vi "ReadConfig.vi"() -> (0 "External Settings":T3)   [LabVIEW 2011]
uses:
  <vilib>/Utility/config.llb/Read Key (I32).vi
  <vilib>/Utility/config.llb/Read Key (U32).vi
  <vilib>/Utility/config.llb/Read Key (String).vi
  <vilib>/Utility/config.llb/Read Key (Path).vi
  <vilib>/Utility/config.llb/NI_LVConfig.lvlib
panel:
  out "Digital Multimeter Card":T1
  out "Matrix version":cluster{"Matrix version":string}
  out "Matrix version":string
  out "Components list":string
  out "Components type":T2
  out "Components type":string
  out "Digital Multimeter":T1
  out "USB Interface":T1
  out "Digital Osciliscope":T1
  out "DC Power Supply":T1
  out "Function Generator":T1
  out "Log":cluster{"Log Level":u32, "Log File":path}
  out "Log File":path
  out "Log Level":u32
  out "Oscilloscope":T4
  out "Global":T5
  out "Timeout":u32
  out "Port":i32
  out "Maximum Delay":i32
  out "Reset Time":i32
  out "Digital Multimeter":T6
  out "Powerline Frequency":u32
  out "Instrument Adress":T7
  out "4072":string
  out "USB":string
  out "5112":string
  out "4110":string
  out "5402":string
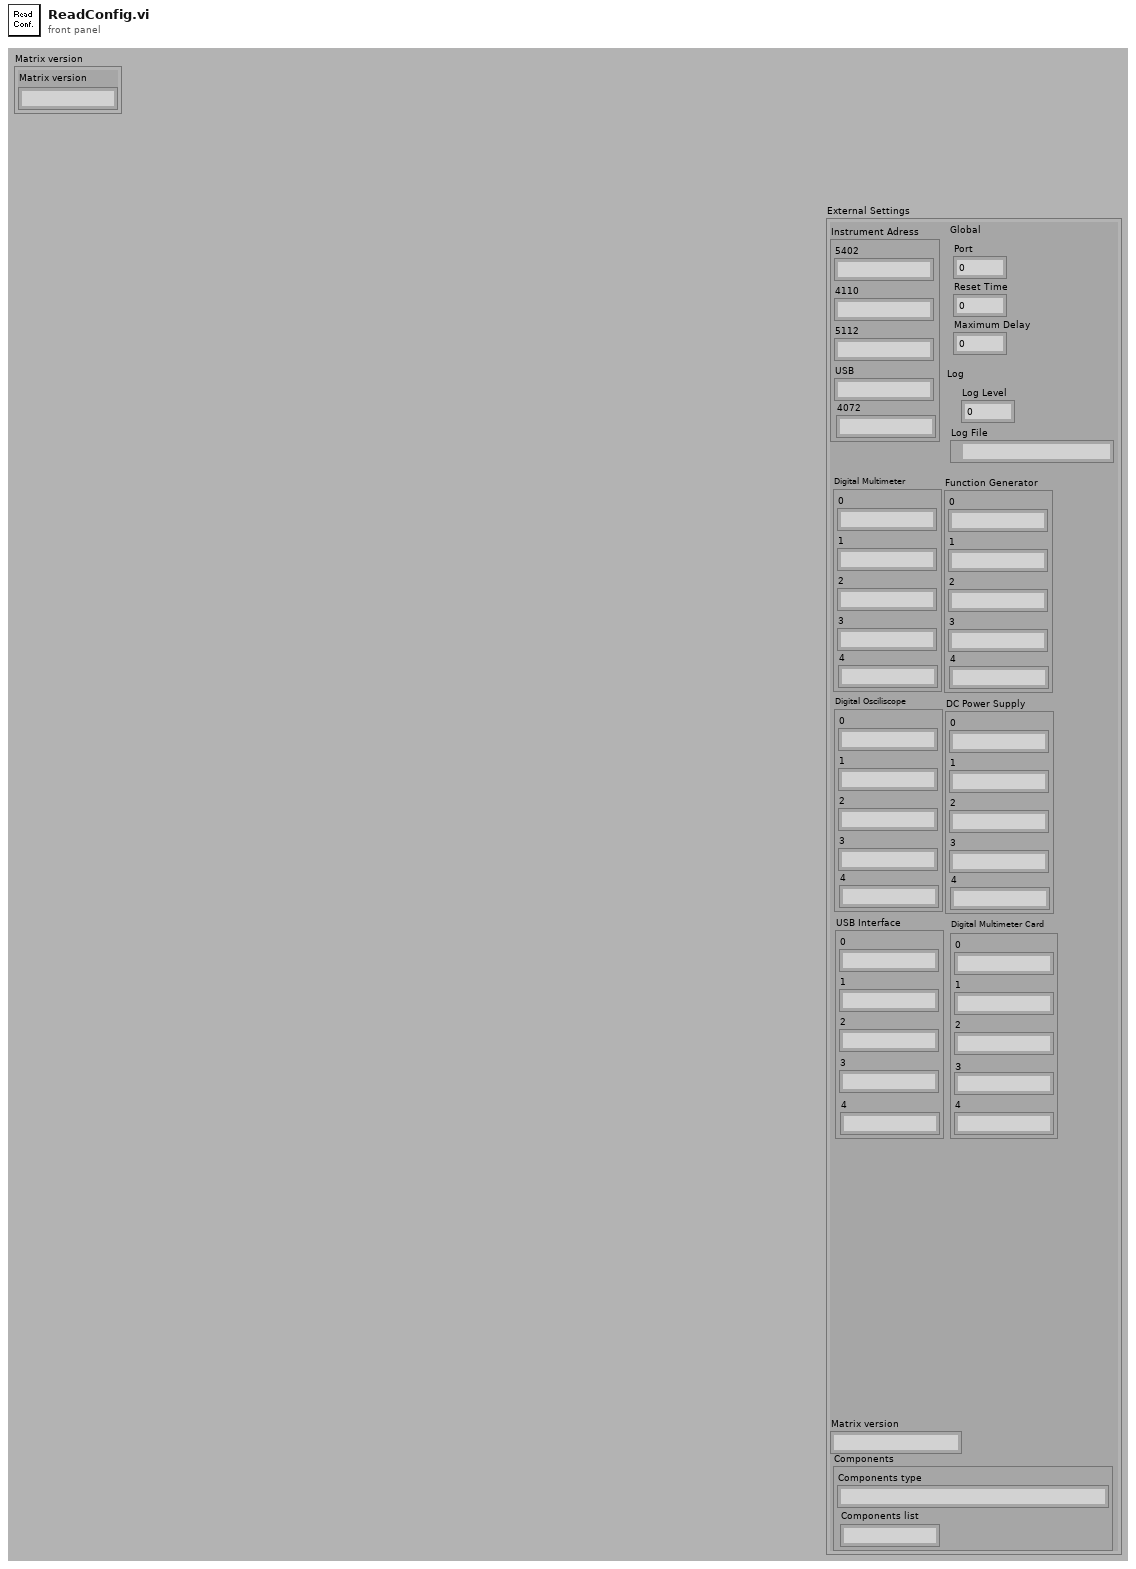
[diagram p1: front panel]
types:
  T1 = cluster{"0":string, "1":string, "2":string, "3":string, "4":string}
  T2 = cluster{"Components type":string, "Components list":string}
  T3 = cluster{"Global":cluster{"Port":i32, "Reset Time":i32, "Maximum Delay":i32}, "Instrument Adress":cluster{"5402":string, "4110":string, "5112":string, "USB":string, "4072":string}, "Log":cluster{"Log Level":u32, "Log File":path}, "Digital Multimeter":cluster{"0":string, "1":string, "2":string, "3":string, "4":string}, "Function Generator":cluster{"0":string, "1":string, "2":string, "3":string, "4":string}, "Digital Osciliscope":cluster{"0":string, "1":string, "2":string, "3":string, "4":string}, "DC Power Supply":cluster{"0":string, "1":string, "2":string, "3":string, "4":string}, "USB Interface":cluster{"0":string, "1":string, "2":string, "3":string, "4":string}, "Components":cluster{"Components type":string, "Components list":string}, "Matrix version":string, "Digital Multimeter Card 2":cluster{"0":string, "1":string, "2":string, "3":string, "4":string}}
  T4 = cluster{"Oscilloscope Board A\nResouce name":string, "Oscilloscope Board B\nResouce name":string, "Additonal Slave Trigger Delay":dbl}
  T5 = cluster{"Port":i32, "Reset Time":i32, "Maximum Delay":i32}
  T6 = cluster{"Powerline Frequency":u32, "Numeric":dbl}
  T7 = cluster{"5401":string, "4110":string, "5112":string, "USB":string, "4072":string}
  T8 = typedef "NI_LVConfig.lvlib/Config Data RefNum.ctl" = refnum<k1>
  T9 = cluster{"[0]":string, "[1]":string, "[2]":string, "[3]":string, "[4]":string}
  T10 = cluster{"Powerline Frequency":u32, "Timeout":u32}
  T11 = cluster{"5402":string, "4110":string, "5112":string, "USB":string, "4072":string}
  T12 = cluster{"Global":cluster{"Port":i32, "Reset Time":i32, "Maximum Delay":i32}, "Instrument Adress":cluster{"5401":string, "4110":string, "5112":string, "USB":string, "4072":string}, "Log":cluster{"Log Level":u32, "Log File":path}, "Digital Multimeter":cluster{"0":string, "1":string, "2":string, "3":string, "4":string}, "Function Generator":cluster{"0":string, "1":string, "2":string, "3":string, "4":string}, "Digital Osciliscope":cluster{"0":string, "1":string, "2":string, "3":string, "4":string}, "DC Power Supply":cluster{"0":string, "1":string, "2":string, "3":string, "4":string}, "USB Interface":cluster{"0":string, "1":string, "2":string, "3":string, "4":string}, "Components type":cluster{"Components type":string, "Components list":string}, "Matrix version":string, "Digital Multimeter Card":cluster{"0":string, "1":string, "2":string, "3":string, "4":string}}
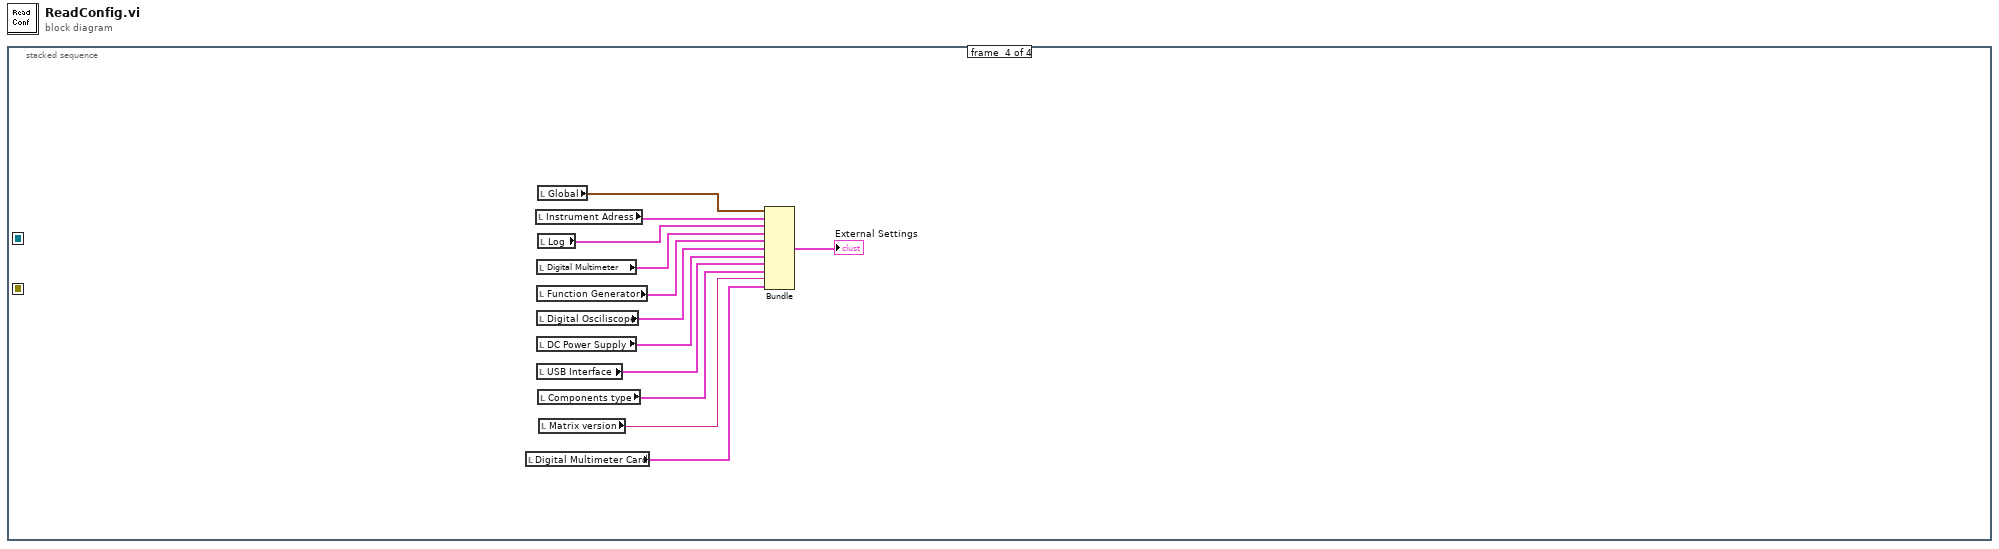
[diagram p0: block diagram]
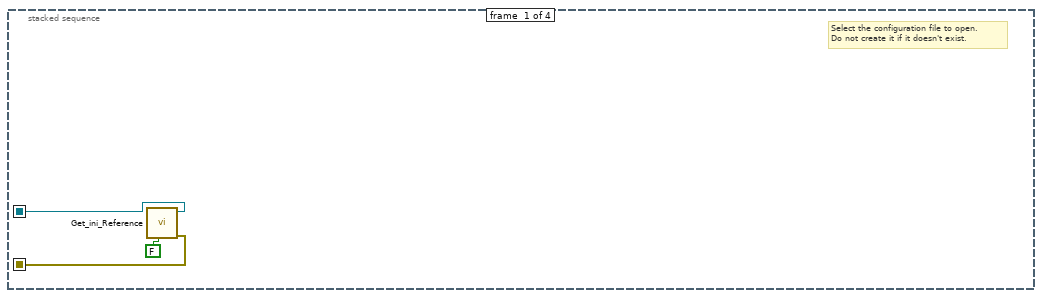
[diagram p2: hidden frame]
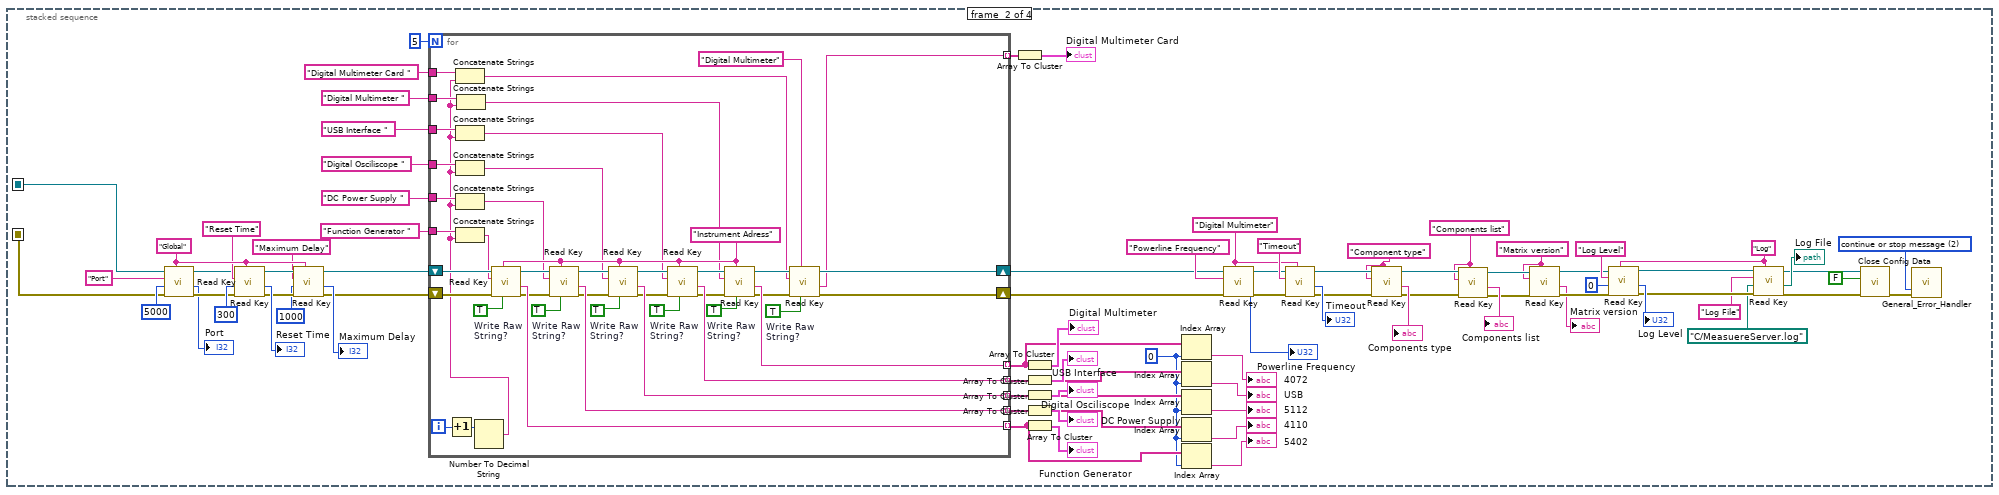
[diagram p3: hidden frame]
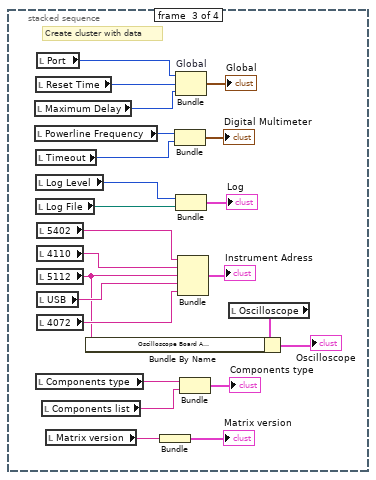
[diagram p4: hidden frame]
diagram:
  n1 = stacked-sequence {
    seq-local: [w2 _ _ _] -> [_ w56 _ _]
    seq-local: [w1 _ _ _] -> [_ w55 _ _]
    frame #0 {
      # "Select the configuration file to open.\nDo not create it if it doesn't exist."
      n2 = call "Get_ini_Reference.vi"("create file if necessary? (T)"=FALSE) -> ("Error out"=w2:errorcluster, "ini Ref"=w1:T8)  [unwired: 8 in, 1 out]
    }
    frame #1 {
      w8 = "Matrix version"
      w10 = "Components list"
      w9 = "Component type"
      w26 = 0
      w46 = "Log"
      w52 = u16 2 items=["no dialog", "OK message", "continue or stop message"] ("type of dialog (OK msg:1)")
      w78 = "Digital Multimeter" ("section")
      w74 = "Global" ("section")
      n3 = call-poly <vilib>:"Read Key.vi"("section"=w74, "error in (no error)"=w56, "default value"=u32 5000, "key"="Port" ("Key 1"), "refnum"=w55) -> ("error out"=w67:errorcluster, "value"=→"Port":i32, "refnum out"=w66:T8)  [unwired: 3 in, 1 out]
      n4 = call-poly <vilib>:"Read Key.vi"("section"=w74, "error in (no error)"=w67, "default value"=300, "key"="Reset Time", "refnum"=w66) -> ("error out"=w73:errorcluster, "value"=→"Reset Time":i32, "refnum out"=w70:T8)  [unwired: 3 in, 1 out]
      n5 = call-poly <vilib>:"Read Key.vi"("section"=w74, "error in (no error)"=w73, "default value"=1000, "key"="Maximum Delay", "refnum"=w70) -> ("error out"=w72:errorcluster, "value"=→"Maximum Delay":i32, "refnum out"=w71:T8)  [unwired: 3 in, 1 out]
      n6 = for {
        N: 5 -> [_]
        tunnel: "Digital Osciliscope " -> [w101]
        tunnel: [w123] -> w31 mode=indexing
        tunnel: [w122] -> w30 mode=indexing
        tunnel: [w121] -> w29 mode=indexing
        tunnel: [w120] -> w28 mode=indexing
        tunnel: [w119] -> w27 mode=indexing
        tunnel: "Digital Multimeter " -> [w105]
        tunnel: "Function Generator " -> [w97]
        tunnel: "DC Power Supply " -> [w100]
        tunnel: "USB Interface " -> [w104]
        shift-right: [w93] -> w39
        shift-left: w72 -> [w126]
        shift-right: [w91] -> w38
        shift-left: w71 -> [w125]
        tunnel: "Digital Multimeter Card " ("section") -> [w87]
        tunnel: [w84] -> w5 mode=indexing
        i -> [w96]
        w90 = TRUE  # Write Raw String?
        w114 = TRUE  # Write Raw String?
        w113 = TRUE  # Write Raw String?
        w112 = TRUE  # Write Raw String?
        w109 = TRUE  # Write Raw String?
        w108 = TRUE  # Write Raw String?
        w124 = "Instrument Adress" ("section")
        n7 = Increment(x=w96) -> (x+1=w95:i32)
        n8 = Number To Decimal String(number=w95) -> (decimal integer string=w88:string)  [unwired: 1 in]
        n9 = Concatenate Strings(w87, w88) -> (w86:string)
        n10 = Concatenate Strings(w104, w88) -> (w103:string)
        n11 = Concatenate Strings(w101, w88) -> (w102:string)
        n12 = Concatenate Strings(w100, w88) -> (w99:string)
        n13 = Concatenate Strings(w97, w88) -> (w98:string)
        n14 = Concatenate Strings(w105, w88) -> (w89:string)
        n15 = call-poly <vilib>:"Read Key.vi"("read raw string? (F)"=w109, "section"=w124, "error in (no error)"=w126, "key"=w98, "refnum"=w125) -> ("error out"=w106:errorcluster, "value"=w123:string, "refnum out"=w107:T8)  [unwired: 3 in, 1 out]
        n16 = call-poly <vilib>:"Read Key.vi"("read raw string? (F)"=w108, "section"=w124, "error in (no error)"=w106, "key"=w99, "refnum"=w107) -> ("error out"=w118:errorcluster, "value"=w122:string, "refnum out"=w117:T8)  [unwired: 3 in, 1 out]
        n17 = call-poly <vilib>:"Read Key.vi"("read raw string? (F)"=w113, "section"=w124, "error in (no error)"=w118, "key"=w102, "refnum"=w117) -> ("error out"=w110:errorcluster, "value"=w121:string, "refnum out"=w111:T8)  [unwired: 3 in, 1 out]
        n18 = call-poly <vilib>:"Read Key.vi"("read raw string? (F)"=w112, "section"=w124, "error in (no error)"=w110, "key"=w103, "refnum"=w111) -> ("error out"=w116:errorcluster, "value"=w120:string, "refnum out"=w115:T8)  [unwired: 3 in, 1 out]
        n19 = call-poly <vilib>:"Read Key.vi"("read raw string? (F)"=w114, "section"=w124, "error in (no error)"=w116, "key"=w89, "refnum"=w115) -> ("error out"=w94:errorcluster, "value"=w119:string, "refnum out"=w92:T8)  [unwired: 3 in, 1 out]
        n20 = call-poly <vilib>:"Read Key.vi"("read raw string? (F)"=w90, "section"="Digital Multimeter", "error in (no error)"=w94, "key"=w86, "refnum"=w92) -> ("error out"=w93:errorcluster, "value"=w84:string, "refnum out"=w91:T8)  [unwired: 3 in, 1 out]
      }
      n21 = Array To Cluster(array=w5) -> (cluster=→"Digital Multimeter Card":T9)
      n22 = Array To Cluster(array=w27) -> (cluster=→"Digital Multimeter":T9)
      n23 = Array To Cluster(array=w28) -> (cluster=→"USB Interface":T9)
      n24 = Array To Cluster(array=w29) -> (cluster=→"Digital Osciliscope":T9)
      n25 = Array To Cluster(array=w30) -> (cluster=→"DC Power Supply":T9)
      n26 = Array To Cluster(array=w31) -> (cluster=→"Function Generator":T9)
      n27 = Index Array(array=w27, index=w26) -> (element=→"4072":string)
      n28 = Index Array(array=w28, index=w26) -> (element=→"USB":string)
      n29 = Index Array(array=w29, index=w26) -> (element=→"5112":string)
      n30 = Index Array(array=w30, index=w26) -> (element=→"4110":string)
      n31 = Index Array(array=w31, index=w26) -> (element=→"5402":string)
      n32 = call-poly <vilib>:"Read Key.vi"("section"=w78, "error in (no error)"=w39, "key"="Powerline Frequency", "refnum"=w38) -> ("error out"=w79:errorcluster, "value"=→"Powerline Frequency":u32, "refnum out"=w80:T8)  [unwired: 4 in, 1 out]
      n33 = call-poly <vilib>:"Read Key.vi"("section"=w78, "error in (no error)"=w79, "key"="Timeout", "refnum"=w80) -> ("error out"=w19:errorcluster, "value"=→"Timeout":u32, "refnum out"=w20:T8)  [unwired: 4 in, 1 out]
      n34 = call-poly <vilib>:"Read Key.vi"("section"=w9, "error in (no error)"=w19, "key"=w9, "refnum"=w20) -> ("error out"=w16:errorcluster, "value"=→"Components type":string, "refnum out"=w17:T8)  [unwired: 4 in, 1 out]
      n35 = call-poly <vilib>:"Read Key.vi"("section"=w10, "error in (no error)"=w16, "key"=w10, "refnum"=w17) -> ("error out"=w12:errorcluster, "value"=→"Components list":string, "refnum out"=w14:T8)  [unwired: 4 in, 1 out]
      n36 = call-poly <vilib>:"Read Key.vi"("section"=w8, "error in (no error)"=w12, "key"=w8, "refnum"=w14) -> ("error out"=w11:errorcluster, "value"=→"Matrix version":string, "refnum out"=w13:T8)  [unwired: 4 in, 1 out]
      n37 = call-poly <vilib>:"Read Key.vi"("section"=w46, "error in (no error)"=w11, "default value"=u32 0, "key"="Log Level", "refnum"=w13) -> ("error out"=w49:errorcluster, "value"=→"Log Level":u32, "refnum out"=w48:T8)  [unwired: 3 in, 1 out]
      n38 = call-poly <vilib>:"Read Key.vi"("section"=w46, "error in (no error)"=w49, "default value"=path "C:/MeasuereServer.log", "key"="Log File", "refnum"=w48) -> ("error out"=w43:errorcluster, "value"=→"Log File":path, "refnum out"=w44:T8)  [unwired: 3 in, 1 out]
      n39 = call <vilib>:"Close Config Data.vi"("error in (no error)"=w43, "write file if changed (T)"=FALSE ("write configuration file? (T)"), "refnum"=w44) -> ("error out"=w53:errorcluster)  [unwired: 7 in, 1 out]
      n40 = call "General_Error_Handler.vi"("type of dialog (OK msg:1)"=w52, "error in (no error)"=w53) -> ()  [unwired: 9 in, 5 out]
    }
    frame #2 {
      # "Create cluster with data"
      n41 = local read "Maximum Delay"() -> (w133:i32)
      n42 = local read "Powerline Frequency"() -> (w146:u32)
      n43 = local read "Reset Time"() -> (w134:i32)
      n44 = local read "Timeout"() -> (w144:u32)
      n45 = local read "Log Level"() -> (w141:u32)
      n46 = local read "Log File"() -> (w140:path)
      n47 = local read "Components type"() -> (w131:string)
      n48 = local read "Port"() -> (w147:i32)
      n49 = local read "5402"() -> (w132:string)
      n50 = local read "4110"() -> (w149:string)
      n51 = local read "5112"() -> (w136:string)
      n52 = local read "USB"() -> (w142:string)
      n53 = local read "4072"() -> (w148:string)
      n54 = local read "Components list"() -> (w129:string)
      n55 = local read "Matrix version"() -> (w127:string)
      n56 = Bundle("Matrix version"=w127) -> (→"Matrix version":cluster{"Matrix version":string})  [unwired: 1 in]
      n57 = Bundle("Powerline Frequency"=w146, "Timeout"=w144) -> (→"Digital Multimeter":T10)  [unwired: 1 in]
      n58 = Bundle "Global"("Port"=w147, "Reset Time"=w134, "Maximum Delay"=w133) -> (→"Global":T5)  [unwired: 1 in]
      n59 = Bundle("Log Level"=w141, "Log File"=w140) -> (→"Log":cluster{"Log Level":u32, "Log File":path})  [unwired: 1 in]
      n60 = Bundle ("Instrument ID")("5402"=w132, "4110"=w149, "5112"=w136, "USB"=w142, "4072"=w148) -> (→"Instrument Adress":T11)  [unwired: 1 in]
      n61 = Bundle("Components type"=w131, "Components list"=w129) -> (→"Components type":T2)  [unwired: 1 in]
      n62 = local read "Oscilloscope"() -> (w137:T4)
      n63 = Bundle By Name(cluster=w137, "Oscilloscope Board A\nResouce name"=w136) -> (→"Oscilloscope":T4)
    }
    frame #3 {
      n64 = local read "Digital Multimeter Card"() -> (w150:T1)
      n65 = local read "Instrument Adress"() -> (w159:T7)
      n66 = local read "Digital Multimeter"() -> (w158:T1)
      n67 = local read "Function Generator"() -> (w157:T1)
      n68 = local read "Digital Osciliscope"() -> (w155:T1)
      n69 = local read "DC Power Supply"() -> (w154:T1)
      n70 = local read "USB Interface"() -> (w156:T1)
      n71 = local read "Global"() -> (w161:T5)
      n72 = local read "Log"() -> (w160:cluster{"Log Level":u32, "Log File":path})
      n73 = local read "Components type"() -> (w153:T2)
      n74 = local read "Matrix version"() -> (w152:string)
      n75 = Bundle("Global"=w161, "Instrument Adress"=w159, "Log"=w160, "Digital Multimeter"=w158, "Function Generator"=w157, "Digital Osciliscope"=w155, "DC Power Supply"=w154, "USB Interface"=w156, "Components type"=w153, "Matrix version"=w152, "Digital Multimeter Card"=w150) -> (→"External Settings":T12)  [unwired: 1 in]
    }
  }
